vi "仪器是否连接判断.vi"(1 "错误输入（无错误）":errorcluster, 2 "元素":string, 3 "VIDPID":string) -> (0 "仪器是否连接":bool)   [LabVIEW 2014]
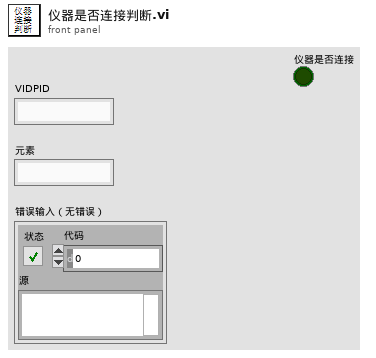
[diagram p1: front panel]
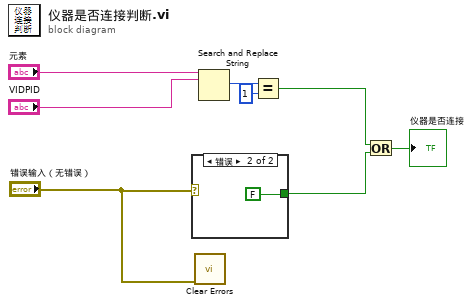
[diagram p0: block diagram]
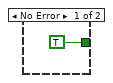
[diagram p2: hidden frame]
diagram:
  n1 = case shown="错误" "错误输入（无错误）" {
    tunnel: [TRUE FALSE] -> w8
    frame No Error {
    }
    frame Error {
    }
  }
  n2 = call <vilib>:"Clear Errors.vi"("error in (no error)"="错误输入（无错误）") -> ()  [unwired: 5 in, 2 out]
  n3 = Search and Replace String(input string="元素", search string="VIDPID") -> (number of replacements=w4:i32)  [unwired: 6 in, 3 out]
  n4 = Equal?(x=w4, y=1) -> (x = y?=w7:bool)
  n5 = Or(x=w7, y=w8) -> (x .or. y?=→"仪器是否连接":bool)
